vi "status_bool_to_color.vi"(6 "status_color_ng":u32(colorbox)=16711680, 7 "status_color_ok":u32(colorbox)=6618880, 8 "status_bool_4":bool=TRUE, 9 "status_bool_3":bool=TRUE, 10 "status_bool_2":bool=TRUE, 11 "status_bool_1":bool=TRUE) -> (3 "status_color":u32)   [LabVIEW 2019]
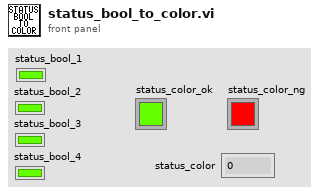
[diagram p1: front panel]
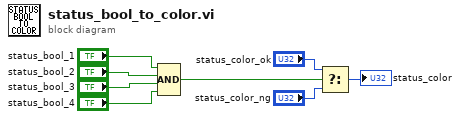
[diagram p0: block diagram]
diagram:
  n1 = Compound Arithmetic op=AND("status_bool_1", "status_bool_2", "status_bool_3", "status_bool_4") -> (w1:bool)
  n2 = Select(t="status_color_ok", s=w1, f="status_color_ng") -> (s? t:f=→"status_color":u32)
